vi "GetProperties.vi"(8 "error in":errorcluster, 11 "Scale in":refnum<class "Scale.lvclass">) -> (0 "error out":errorcluster, 3 "Scale out":refnum<class "Scale.lvclass">)   [LabVIEW 2014, in "Raspberry Pi Compatible Compiler for LabVIEW.lvlib" / "Scale.lvclass"]
uses:
  Scale.lvclass
  Scale.lvclass/Scale.ctl
  GObject/GObject.lvclass
  Text/Text.lvclass
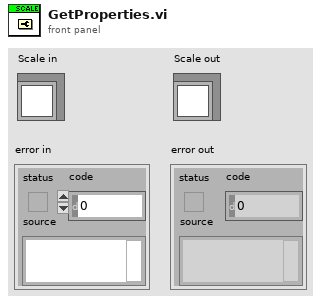
[diagram p1: front panel]
types:
  T1 = typedef "LVFormatAndPrecisionTypeDef.ctl" = cluster{"Format":u8, "Precision":u8}
  T2 = typedef "LVTextColorsTypeDef.ctl" = cluster{"Text Color":u32, "Background Color":u32}
  T3 = typedef "LVRangeTypeDef.ctl" = cluster{"Minimum":dbl, "Maximum":dbl, "Increment":dbl, "Minor Increment":dbl, "Start":dbl}
  T4 = typedef "LVTickColorsTypeDef.ctl" = cluster{"Tick Color":u32, "Minor Tick Color":u32}
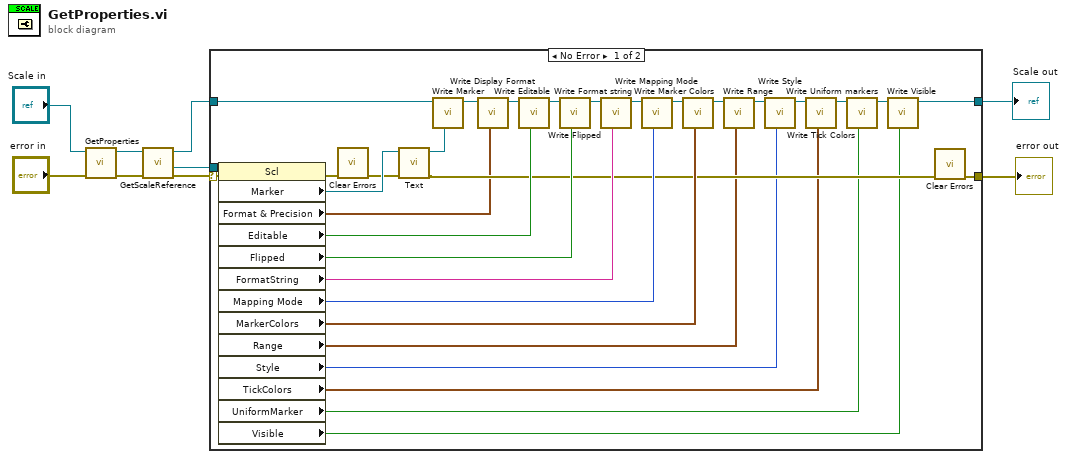
[diagram p0: block diagram]
diagram:
  n1 = call-parent "GetProperties.vi"("error in"="error in", "GObject in"="Scale in") -> ("error out"=w6:errorcluster, "GObject out"=w7:refnum<class "Scale.lvclass">)  [unwired: 8 in]
  n2 = call "GetScaleReference.vi"("error in"=w6, "Scale in"=w7) -> ("error out"=w5:errorcluster, "scale reference"=w4:refnum<vi>, "Scale out"=w3:refnum<class "Scale.lvclass">)  [unwired: 7 in]
  n3 = case shown="No Error" w5 {
    selector: w5 -> [w41 w42]
    tunnel: w4 -> [w40 _]
    tunnel: w3 -> [w20 w43]
    tunnel: [w30 w43] -> w2
    tunnel: [w12 w42] -> w1
    frame No Error {
      n4 = property class="Scl"(reference=w40, error in=w41) -> (error out=w23:errorcluster, "Marker"=w18:refnum<vi>, "Format & Precision"=w11:T1, "Editable"=w29:bool, "Flipped"=w28:bool, "FormatString"=w27:string, "Mapping Mode"=w26:u8, "MarkerColors"=w25:T2, "Range"=w17:T3, "Style"=w16:u8, "TickColors"=w15:T4, "UniformMarker"=w14:bool, "Visible"=w13:bool)  [unwired: 1 out]
      n5 = call <vilib>:"Clear Errors.vi"("error in (no error)"=w23) -> ("error out"=w10:errorcluster)  [unwired: 5 in, 1 out]
      n6 = call "Text.vi"("error in"=w10, "Gen Refnum"=w18) -> ("error out"=w22:errorcluster, "Text out"=w19:refnum<class "Text.lvclass">)  [unwired: 8 in]
      n7 = call "Write Marker.vi"("Marker"=w19, "Scale in"=w20) -> ("Scale out"=w21:refnum<class "Scale.lvclass">)  [unwired: 7 in]
      n8 = call "Write Display Format.vi"("Display Format"=w11, "Scale in"=w21) -> ("Scale out"=w39:refnum<class "Scale.lvclass">)  [unwired: 7 in]
      n9 = call "Write Editable.vi"("Editable"=w29, "Scale in"=w39) -> ("Scale out"=w38:refnum<class "Scale.lvclass">)  [unwired: 7 in]
      n10 = call "Write Flipped.vi"("Flipped"=w28, "Scale in"=w38) -> ("Scale out"=w37:refnum<class "Scale.lvclass">)  [unwired: 7 in]
      n11 = call "Write Format string.vi"("Format string"=w27, "Scale in"=w37) -> ("Scale out"=w36:refnum<class "Scale.lvclass">)  [unwired: 7 in]
      n12 = call "Write Mapping Mode.vi"("Mapping Mode"=w26, "Scale in"=w36) -> ("Scale out"=w35:refnum<class "Scale.lvclass">)  [unwired: 7 in]
      n13 = call "Write Marker Colors.vi"("Marker Colors"=w25, "Scale in"=w35) -> ("Scale out"=w24:refnum<class "Scale.lvclass">)  [unwired: 7 in]
      n14 = call "Write Range.vi"("Range"=w17, "Scale in"=w24) -> ("Scale out"=w34:refnum<class "Scale.lvclass">)  [unwired: 7 in]
      n15 = call "Write Style.vi"("Style"=w16, "Scale in"=w34) -> ("Scale out"=w33:refnum<class "Scale.lvclass">)  [unwired: 7 in]
      n16 = call "Write Tick Colors.vi"("Tick Colors"=w15, "Scale in"=w33) -> ("Scale out"=w32:refnum<class "Scale.lvclass">)  [unwired: 7 in]
      n17 = call "Write Uniform markers.vi"("Uniform markers"=w14, "Scale in"=w32) -> ("Scale out"=w31:refnum<class "Scale.lvclass">)  [unwired: 7 in]
      n18 = call "Write Visible.vi"("Visible"=w13, "Scale in"=w31) -> ("Scale out"=w30:refnum<class "Scale.lvclass">)  [unwired: 7 in]
      n19 = call <vilib>:"Clear Errors.vi"("error in (no error)"=w22) -> ("error out"=w12:errorcluster)  [unwired: 5 in, 1 out]
    }
    frame Error {
    }
  }
  "error out" <- w1
  "Scale out" <- w2
